vi "Grubbs_Test Sub.vi"(6 "Уровень значимости":dbl, 7 "Исходная выборка":dbl[](graph)) -> (0 "СКО":dbl, 1 "Среднее":dbl, 2 "Array":dbl[](array[numeric]), 3 "Обработанные результаты":dbl[](graph))   [LabVIEW 2013]
uses:
  Grubbs_Test_States.ctl
  <vilib>/Analysis/NI_AALBase.lvlib
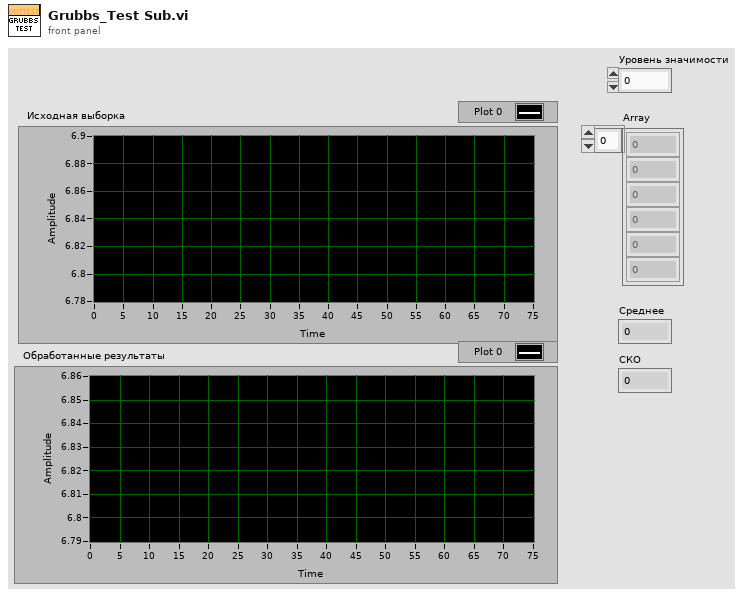
[diagram p1: front panel]
types:
  T1 = typedef "Grubbs_Test_States.ctl" = enum16{"Инициализация", "Расчет ошибок", "Проверка на промахи", "Завершение работы"}
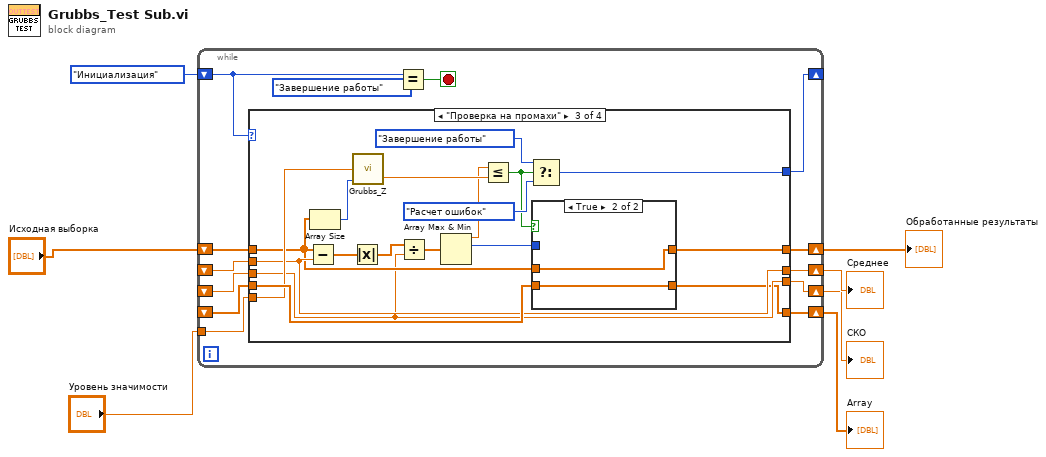
[diagram p0: block diagram]
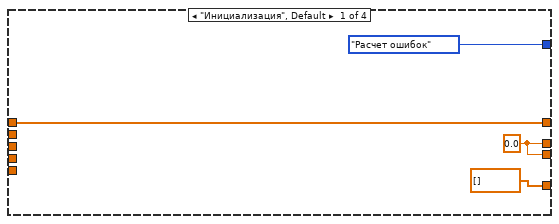
[diagram p2: hidden frame]
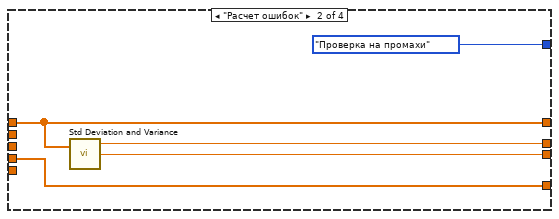
[diagram p3: hidden frame]
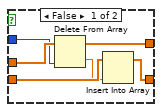
[diagram p4: hidden frame]
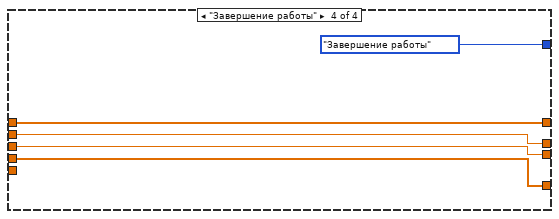
[diagram p5: hidden frame]
diagram:
  n1 = while {
    shift-right: [w20] -> _
    shift-left: Grubbs_Test_States."Инициализация" -> [w18]
    shift-right: [w13] -> w3
    shift-left: "Исходная выборка" -> [w14]
    shift-right: [w8] -> w6
    shift-left: _ -> [w10]
    shift-right: [w16] -> w5
    shift-left: _ -> [w9]
    shift-right: [w12] -> w2
    shift-left: _ -> [w11]
    tunnel: "Уровень значимости" -> [w15]
    stop <- w17 stop-if-true
    n2 = case shown="\"Проверка на промахи\"" w18 {
      tunnel: [Grubbs_Test_States."Расчет ошибок" Grubbs_Test_States."Проверка на промахи" w43 Grubbs_Test_States."Завершение работы"] -> w20
      tunnel: [w23 w26 w35 w58] -> w16
      tunnel: w15 -> [_ _ w39 _]
      tunnel: [w22 w28 w31 w60] -> w13
      tunnel: w14 -> [w22 w28 w36 w60]
      tunnel: [dbl[] [] w29 w30 w57] -> w12
      tunnel: w11 -> [_ w29 w47 w57]
      tunnel: w10 -> [_ _ w37 w59]
      tunnel: w9 -> [_ _ w35 w58]
      tunnel: [w23 w27 w37 w59] -> w8
      frame "Инициализация", Default {
        w23 = 0.0
      }
      frame "Расчет ошибок" {
        n3 = call <vilib>:"Std Deviation and Variance.vi"("X"=w28) -> ("mean"=w27:dbl, "standard deviation"=w26:dbl)  [unwired: 1 in, 1 out]
      }
      frame "Проверка на промахи" {
        n4 = Subtract(x=w36, y=w37) -> (x-y=w38:dbl[])
        n5 = Array Size(array=w36) -> (size(s)=w40:i32)
        n6 = Absolute Value(x=w38) -> (abs(x)=w46:dbl[])
        n7 = call "Grubbs_Z.vi"("n"=w40, "q"=w39) -> ("G"=w41:dbl)  [unwired: 2 in]
        n8 = Divide(x=w46, y=w35) -> (x/y=w34:dbl[])
        n9 = Array Max & Min(array=w34) -> (max value=w33:dbl, max index (indices)=w32:i32)  [unwired: 2 out]
        n10 = Less Or Equal?(x=w33, y=w41) -> (x <= y?=w42:bool)
        n11 = Select(t=Grubbs_Test_States."Завершение работы", s=w42, f=Grubbs_Test_States."Расчет ошибок") -> (s? t:f=w43:T1)
        n12 = case shown="True" w42 {
          tunnel: w36 -> [w53 w55]
          tunnel: [w52 w55] -> w31
          tunnel: w47 -> [w51 w54]
          tunnel: [w50 w54] -> w30
          tunnel: w32 -> [w48 _]
          frame False {
            n13 = Delete From Array(array=w53, index=w48) -> (deleted portion=w49:dbl, array with subset deleted=w52:dbl[])  [unwired: 1 in]
            n14 = Insert Into Array(array=w51, new element=w49) -> (w50:dbl[])  [unwired: 1 in]
          }
          frame True {
          }
        }
      }
      frame "Завершение работы" {
      }
    }
    n15 = Equal?(x=w18, y=Grubbs_Test_States."Завершение работы") -> (x = y?=w17:bool)
  }
  "Array" <- w2
  "Среднее" <- w6
  "СКО" <- w5
  "Обработанные результаты" <- w3
